vi "Rcv Cmd.vi"(8 "error in":errorcluster, 11 "tCRD in":refnum<class "Aircraft OPCCRD.lvclass">) -> (0 "error out":errorcluster, 3 "tCRD out":refnum<class "Aircraft OPCCRD.lvclass">)   [LabVIEW 2015, in "Aircraft OPCCRD.lvclass"]
uses:
  Aircraft OPCCRD.lvclass
  Aircraft OPCCRD.lvclass/Aircraft OPCCRD.ctl
  Reusable/File IO/Class/File Observer.lvclass/File Observer.ctl
  Reusable/Instrument/state.ctl
  <vilib>/Utility/error.llb/Error Cluster From Error Code.vi
  <vilib>/rvi/errors/niLvFpgaAdjustHostInterfaceError.vi
  <vilib>/rvi/interface/nirviReadWriteControl/nirviReadWriteControl.xnode
  tFPGA Ref.ctl
  FPGA Bitfiles/Aircraft OPCRD Server.lvbitx
  File Observer/Tim File Observer.lvclass
  Reusable/File IO/Class/File Observer.lvclass
  Reusable/Instrument/Instrument.lvclass
  Reusable/CRDS/Main/CRDS.lvclass
  NiFpgaLv.dll
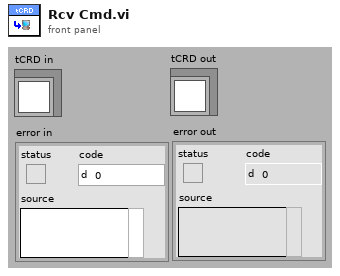
[diagram p1: front panel]
types:
  T1 = typedef "Instrument.lvclass/state.ctl" = enum8{"Configure", "Acquire", "Wait", "Quit", "Handle Error", "NOOP"}
  T2 = typedef "Aircraft OPCCRD.lvclass/tFPGA Ref.ctl" = refnum<k20>
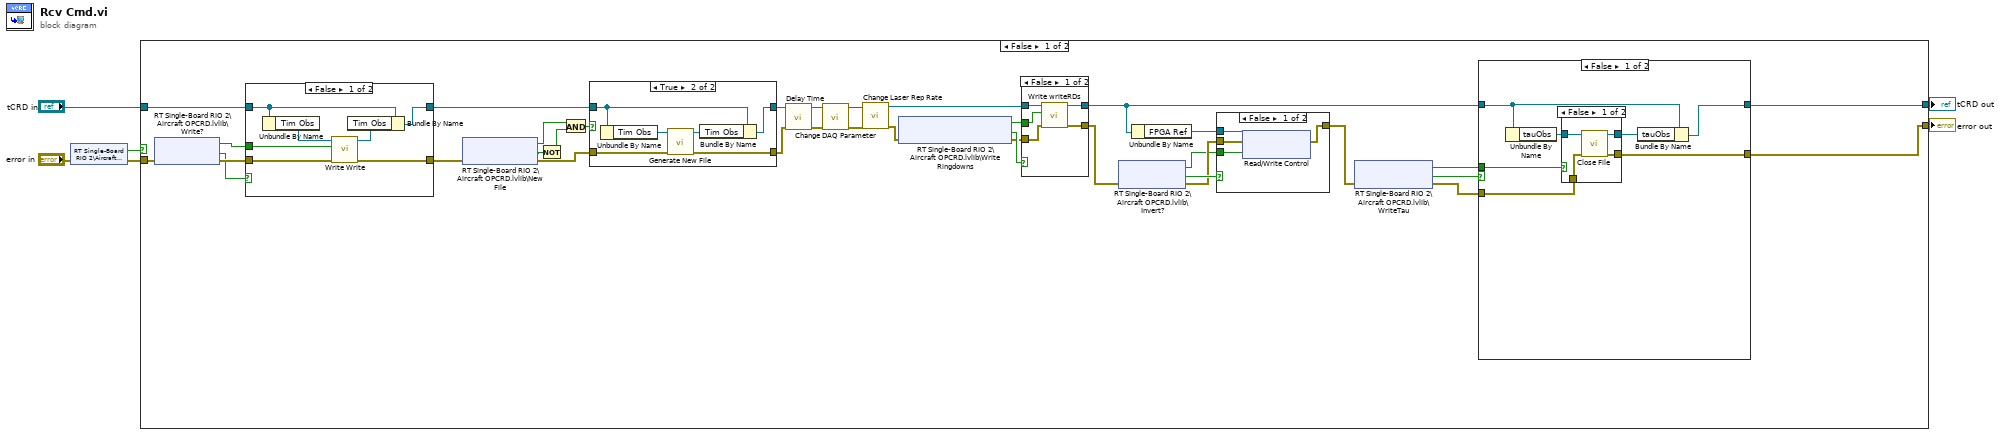
[diagram p0: block diagram]
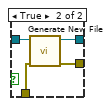
[diagram p2: hidden frame]
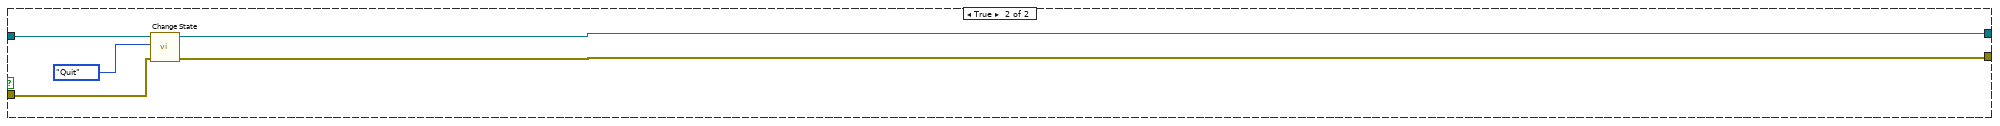
[diagram p8: hidden frame]
diagram:
  n1 = shared-variable "RT Single-Board RIO 2\\Aircraft OPCRD.lvlib\\Stop"(error in="error in") -> (w6:bool, error out=w3:errorcluster)
  n2 = case shown="False" w6 {
    tunnel: "tCRD in" -> [w41 w92]
    tunnel: w3 -> [w35 w90]
    tunnel: [w9 w89] -> w2
    tunnel: [w11 w88] -> w1
    frame False {
      n3 = shared-variable "RT Single-Board RIO 2\\Aircraft OPCRD.lvlib\\Write?"(error in=w35) -> (w39:bool, error out=w40:errorcluster, w38:bool)  [unwired: 1 in]
      n4 = case shown="False" w38 {
        tunnel: w41 -> [w83 w87]
        tunnel: [w82 w87] -> w28
        tunnel: w40 -> [w81 w86]
        tunnel: [w80 w86] -> w29
        tunnel: w39 -> [w79 _]
        frame False {
          n5 = Unbundle By Name(w83) -> ("Tim Obs"=w85:refnum<class "Tim File Observer.lvclass">)
          n6 = call "Write Write.vi"("error in (no error)"=w81, "Write"=w79, "File Observer in"=w85) -> ("error out"=w80:errorcluster, "File Observer out"=w84:refnum<class "Tim File Observer.lvclass">)  [unwired: 7 in]
          n7 = Bundle By Name(cluster=w83, "Tim Obs"=w84) -> (w82:refnum<class "Aircraft OPCCRD.lvclass">)
        }
        frame True {
        }
      }
      n8 = shared-variable "RT Single-Board RIO 2\\Aircraft OPCRD.lvlib\\New File"(error in=w29) -> (w22:bool, error out=w26:errorcluster, w21:bool)  [unwired: 1 in]
      n9 = Not(x=w21) -> (.not. x?=w20:bool)
      n10 = And(x=w22, y=w20) -> (x .and. y?=w19:bool)
      n11 = case shown="True" w19 {
        tunnel: w28 -> [w65 w70]
        tunnel: [w65 w68] -> w27
        tunnel: w26 -> [w64 w67]
        tunnel: [w64 w66] -> w25
        frame False {
        }
        frame True {
          n12 = Unbundle By Name(w70) -> ("Tim Obs"=w71:refnum<class "Tim File Observer.lvclass">)
          n13 = call-dynamic "Generate New File.vi"("error in"=w67, "File Obs in"=w71) -> ("error out"=w66:errorcluster, "File Obs out"=w69:refnum<class "Tim File Observer.lvclass">)  [unwired: 7 in, 1 out]
          n14 = Bundle By Name(cluster=w70, "Tim Obs"=w69) -> (w68:refnum<class "Aircraft OPCCRD.lvclass">)
        }
      }
      n15 = call "Delay Time.vi"("error in"=w25, "tCRD in"=w27) -> ("error out"=w36:errorcluster, "tCRD out"=w37:refnum<class "Aircraft OPCCRD.lvclass">)  [unwired: 8 in]
      n16 = call "Change DAQ Parameter.vi"("error in"=w36, "tCRD in"=w37) -> ("error out"=w32:errorcluster, "tCRD out"=w33:refnum<class "Aircraft OPCCRD.lvclass">)  [unwired: 8 in]
      n17 = call "Change Laser Rep Rate.vi"("error in"=w32, "tCRD in"=w33) -> ("error out"=w24:errorcluster, "tCRD out"=w34:refnum<class "Aircraft OPCCRD.lvclass">)  [unwired: 8 in]
      n18 = shared-variable "RT Single-Board RIO 2\\Aircraft OPCRD.lvlib\\Write Ringdowns"(error in=w24) -> (w31:bool, error out=w23:errorcluster, w30:bool)  [unwired: 1 in]
      n19 = case shown="False" w30 {
        tunnel: w34 -> [w76 w78]
        tunnel: [w75 w78] -> w8
        tunnel: [w74 w77] -> w7
        tunnel: w23 -> [w73 w77]
        tunnel: w31 -> [w72 _]
        frame False {
          n20 = call "Write writeRDs.vi"("error in"=w73, "Write?"=w72, "CRDS in"=w76) -> ("error out"=w74:errorcluster, "CRDS out"=w75:refnum<class "Aircraft OPCCRD.lvclass">)  [unwired: 7 in]
        }
        frame True {
        }
      }
      n21 = shared-variable "RT Single-Board RIO 2\\Aircraft OPCRD.lvlib\\Invert?"(error in=w7) -> (w15:bool, error out=w16:errorcluster, w17:bool)  [unwired: 1 in]
      n22 = Unbundle By Name(w8) -> ("FPGA Ref"=w18:T2)
      n23 = case shown="False" w17 {
        tunnel: w18 -> [w62 _]
        tunnel: w16 -> [w61 w63]
        tunnel: [w60 w63] -> w14
        tunnel: w15 -> [w59 _]
        frame False {
          n24 = xnode "Read/Write Control"("FPGA VI Reference In"=w62, "error in"=w61, "InvertLaser?"=w59) -> ("error out"=w60:errorcluster)  [unwired: 1 out]
        }
        frame True {
        }
      }
      n25 = shared-variable "RT Single-Board RIO 2\\Aircraft OPCRD.lvlib\\WriteTau"(error in=w14) -> (w12:bool, error out=w10:errorcluster, w13:bool)  [unwired: 1 in]
      n26 = case shown="False" w13 {
        tunnel: w12 -> [w48 _]
        tunnel: w8 -> [w46 w58]
        tunnel: [w45 w58] -> w11
        tunnel: w10 -> [w43 w57]
        tunnel: [w42 w57] -> w9
        frame False {
          n27 = Unbundle By Name(w46) -> ("tauObs"=w47:refnum<class "File Observer.lvclass">)
          n28 = case shown="False" w48 {
            tunnel: w47 -> [w52 w56]
            tunnel: [w51 w55] -> w44
            tunnel: w43 -> [w50 w54]
            tunnel: [w49 w53] -> w42
            frame False {
              n29 = call-dynamic "Close File.vi"("error in"=w50, "File Obs in"=w52) -> ("error out"=w49:errorcluster, "File Obs out"=w51:refnum<class "File Observer.lvclass">)  [unwired: 8 in]
            }
            frame True {
              n30 = call-dynamic "Generate New File.vi"("error in"=w54, "File Obs in"=w56) -> ("error out"=w53:errorcluster, "File Obs out"=w55:refnum<class "File Observer.lvclass">)  [unwired: 7 in, 1 out]
            }
          }
          n31 = Bundle By Name(cluster=w46, "tauObs"=w44) -> (w45:refnum<class "Aircraft OPCCRD.lvclass">)
        }
        frame True {
        }
      }
    }
    frame True {
      n32 = call "Change State.vi"("error in"=w90, "instr state"=state."Quit", "Instrument in"=w92) -> ("error out"=w89:errorcluster, "Instrument out"=w88:refnum<class "Aircraft OPCCRD.lvclass">)  [unwired: 7 in]
    }
  }
  "error out" <- w2
  "tCRD out" <- w1
